vi "Destroy.vi"(8 "error in (no error)":errorcluster, 11 "Float64 in":refnum<class "Float64.lvclass">) -> (0 "error out":errorcluster)   [LabVIEW 2015, in "MDSplus.lvlib" / "Float64.lvclass"]
uses:
  Float64.lvclass
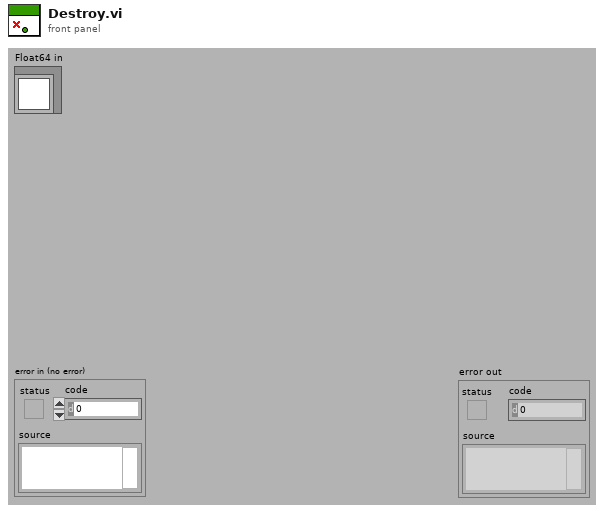
[diagram p1: front panel]
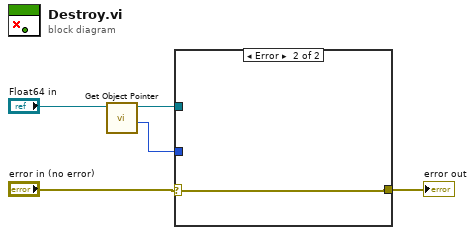
[diagram p0: block diagram]
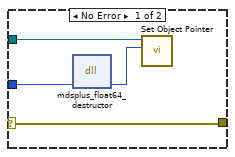
[diagram p2: hidden frame]
diagram:
  n1 = call-dynamic "Get Object Pointer.vi"("Data in"="Float64 in") -> ("Object Pointer"=w4:i64, "Data out"=w5:refnum<class "Float64.lvclass">)  [unwired: 8 in, 1 out]
  n2 = case shown="Error" "error in (no error)" {
    selector: "error in (no error)" -> [w6 w10]
    tunnel: w5 -> [w9 _]
    tunnel: w4 -> [w8 _]
    tunnel: [w6 w10] -> w2
    frame No Error {
      n3 = dll-call lib="MDSobjectsLVShr" fn="mdsplus_float64_destructor"("lvFloat64Ptr"=w8) -> ("lvFloat64Ptr"=w7:i64)  [unwired: 4 in, 2 out]
      n4 = call-dynamic "Set Object Pointer.vi"("Object Pointer"=w7, "Data in"=w9) -> ()  [unwired: 9 in, 1 out]
    }
    frame Error {
    }
  }
  "error out" <- w2
